vi "Meas 2 Target.vi"(10 "LBCB  Data":T1[](array[typedef]), 11 "Target":T2) -> (3 "Measured Value":T2)   [LabVIEW 2013]
uses:
  MixedMode/Messages/Target.ctl
  Data Access Objects/Metadata/LBCB Number.ctl
  MixedMode/Mixed Mode Cartesian Data.ctl
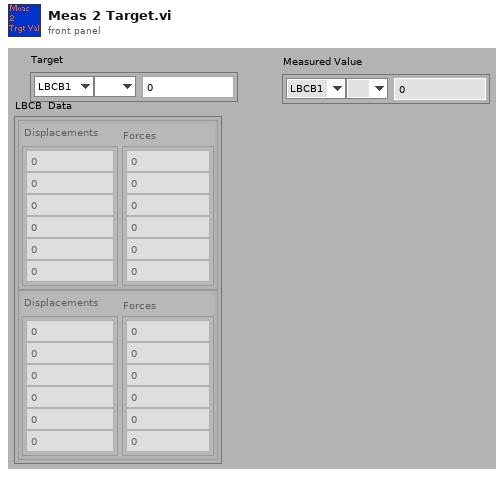
[diagram p1: front panel]
types:
  T1 = typedef "Mixed Mode Cartesian Data.ctl" = cluster{"Displacements":dbl[], "Forces":dbl[]}
  T2 = typedef "Target.ctl" = cluster{"LBCB Number":T3, "DOF Vectors":enum16{" ", "Dx", "Dy", "Dz", "Rx", "Ry", "Rz", "Fx", "Fy", "Fz", "Mx", "My", "Mz"}, "Amount":dbl}
  T3 = typedef "LBCB Number.ctl" = enum16{"LBCB1", "LBCB2"}
  T4 = enum16{" ", "Dx", "Dy", "Dz", "Rx", "Ry", "Rz", "Fx", "Fy", "Fz", "Mx", "My", "Mz"}
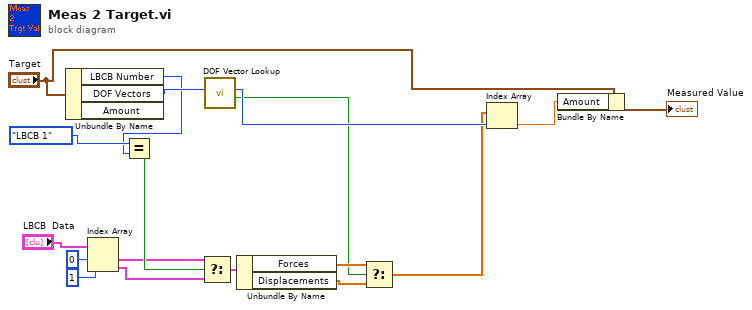
[diagram p0: block diagram]
diagram:
  n1 = Unbundle By Name("Target") -> ("LBCB Number"=w7:T3, "DOF Vectors"=w18:T4)  [unwired: 1 out]
  n2 = Index Array(array="LBCB  Data", index #1=0 ("index"), index #2=1 ("index")) -> (element #1=w6:T1, element #2=w2:T1)
  n3 = Equal?(x=enum16{"LBCB 1", "LBCB 2"}."LBCB 1", y=w7) -> (x = y?=w17:bool)
  n4 = Select(t=w6, s=w17, f=w2) -> (s? t:f=w13:T1)
  n5 = call "DOF Vector Lookup.vi"("DOF Vectors"=w18) -> ("IsForce"=w8:bool, "Index"=w14:u32)  [unwired: 9 out]
  n6 = Unbundle By Name(w13) -> ("Forces"=w12:dbl[], "Displacements"=w11:dbl[])
  n7 = Select(t=w12, s=w8, f=w11) -> (s? t:f=w1:dbl[])
  n8 = Index Array(array=w1, index=w14) -> (element=w10:dbl)
  n9 = Bundle By Name(cluster="Target", "Amount"=w10) -> (→"Measured Value":T2)
